vi "ConfigXMLCore.vi"(9 "ConnectionData":T1, 10 "controlsToSave":refnum<vi>[](array[refnum]), 11 "ConfigXMLControl":T2) -> ()   [LabVIEW 2016]
uses:
  ConfigXMLControl.ctl
  General/CorePluginInfo.ctl
  General/RemoteFiles/connectionData.ctl
  <vilib>/Rock Robotics/Network Tables/NT Read String.vi
panel:
  # "Core controller VI for the XML config plugin.\nhandles all saving, loading, file transfer, etc."
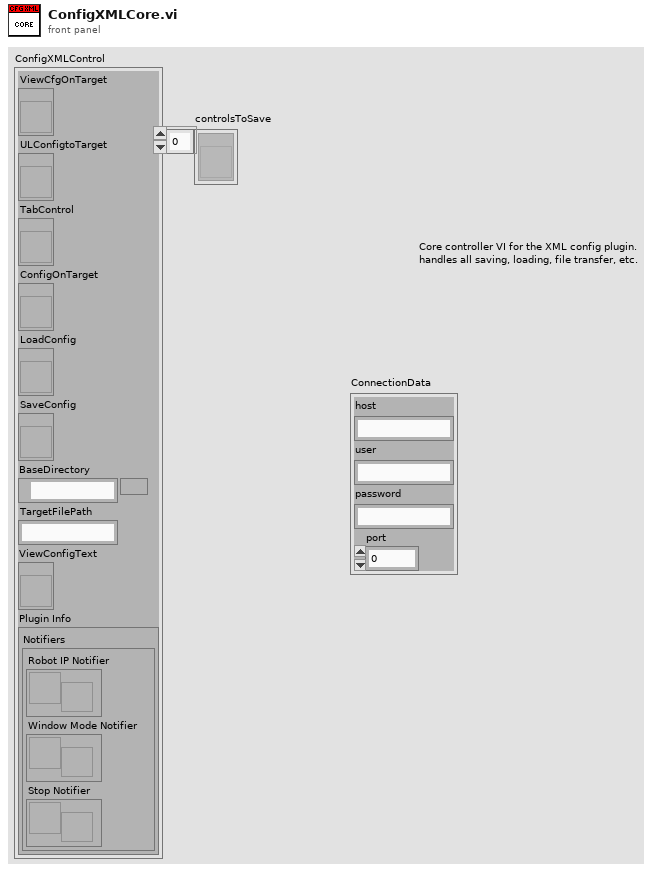
[diagram p1: front panel]
types:
  T1 = typedef "connectionData.ctl" = cluster{"host":string, "user":string, "password":string, "port":u16}
  T2 = typedef "ConfigXMLControl.ctl" = cluster{"ViewCfgOnTarget":refnum<vi>, "ULConfigtoTarget":refnum<vi>, "TabControl":refnum<vi>, "ConfigOnTarget":refnum<vi>, "LoadConfig":refnum<vi>, "SaveConfig":refnum<vi>, "BaseDirectory":path, "TargetFilePath":string, "ViewConfigText":refnum<vi>, "Plugin Info":T3}
  T3 = typedef "CorePluginInfo.ctl" = cluster{"Notifiers":cluster{"Robot IP Notifier":refnum<notifier>, "Window Mode Notifier":refnum<notifier>, "Stop Notifier":refnum<notifier>}}
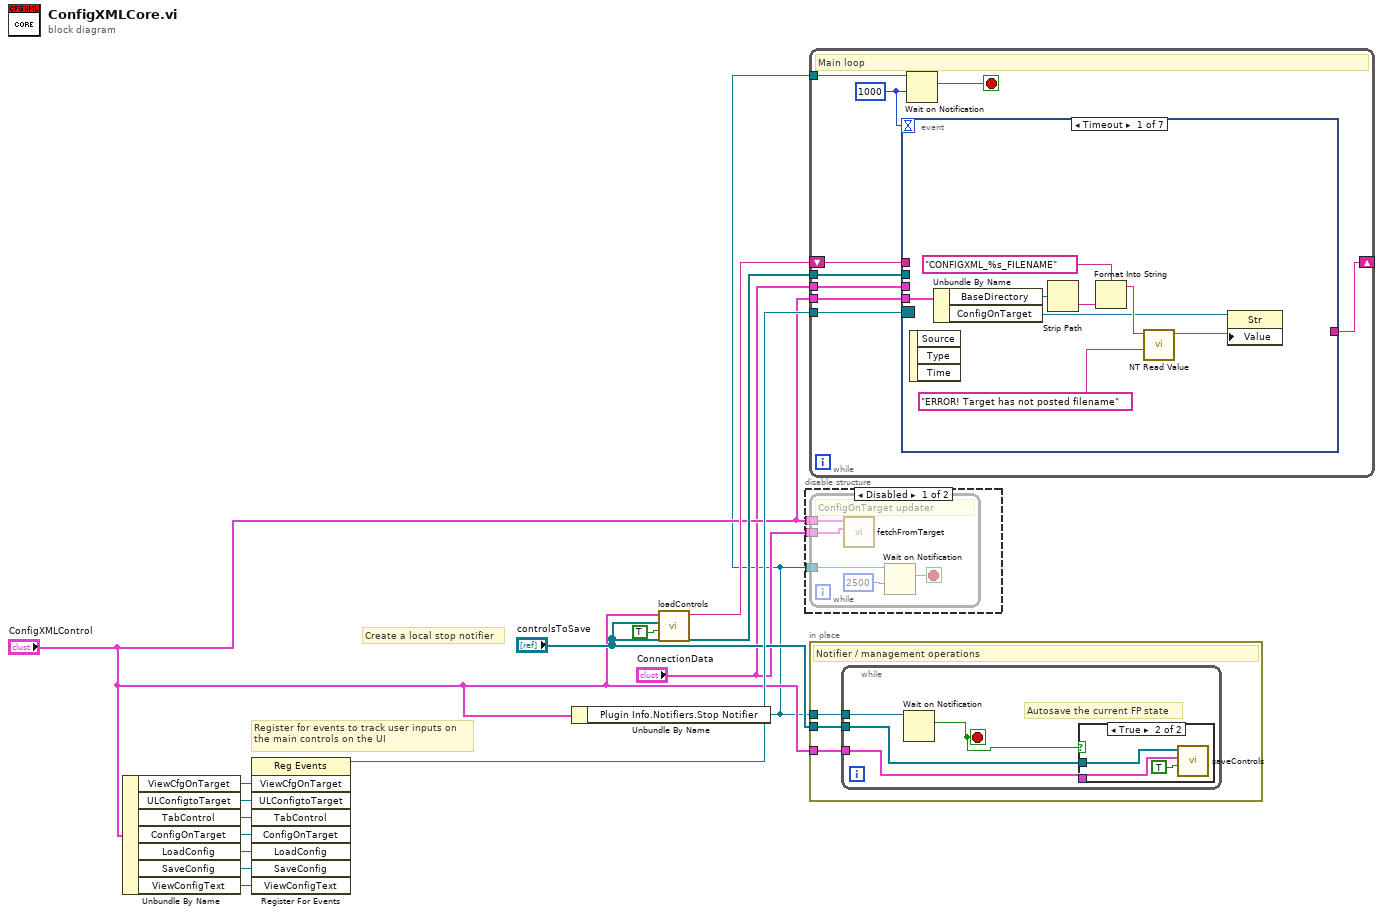
[diagram p0: block diagram]
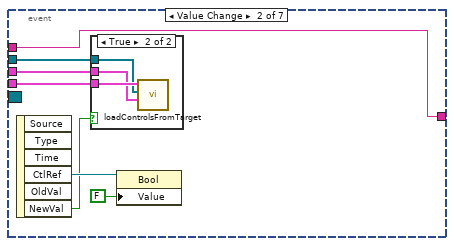
[diagram p3: hidden frame]
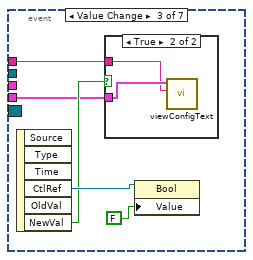
[diagram p5: hidden frame]
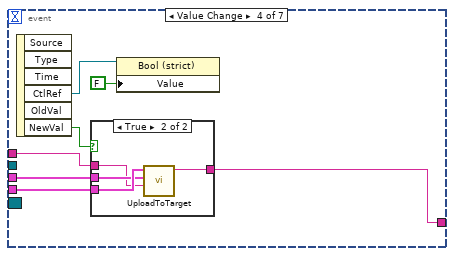
[diagram p7: hidden frame]
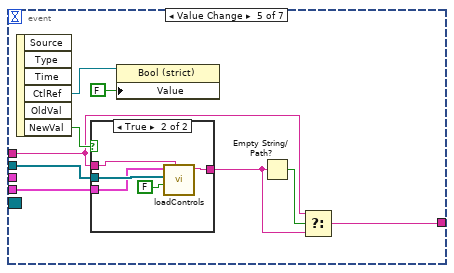
[diagram p9: hidden frame]
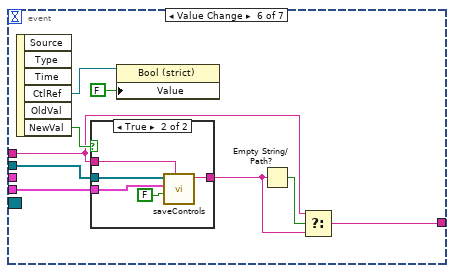
[diagram p11: hidden frame]
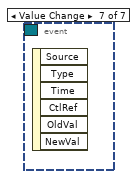
[diagram p13: hidden frame]
diagram:
  # "Create a local stop notifier"
  # "Register for events to track user inputs on\nthe main controls on the UI"
  n1 = Unbundle By Name("ConfigXMLControl") -> ("ViewCfgOnTarget"=w14:refnum<vi>, "ULConfigtoTarget"=w13:refnum<vi>, "TabControl"=w12:refnum<vi>, "ConfigOnTarget"=w11:refnum<vi>, "LoadConfig"=w10:refnum<vi>, "SaveConfig"=w9:refnum<vi>, "ViewConfigText"=w2:refnum<vi>)
  n2 = register-events(w14, w13, w12, w11, w10, w9, w2) -> (reference out=w8:refnum<event-registration>)  [unwired: 2 in, 1 out]
  n3 = Unbundle By Name("ConfigXMLControl") -> ("Plugin Info.Notifiers.Stop Notifier"=w1:refnum<notifier>)
  n4 = call "loadControls.vi"("Autoload?"=TRUE, "ControlsToLoad"="controlsToSave", "ConfigXMLControls"="ConfigXMLControl") -> ("nameUsed"=w6:string)  [unwired: 7 in, 1 out]
  n5 = disable-structure shown="Disabled" {
    disable-tunnel: "ConfigXMLControl" -> [w17 _]
    disable-tunnel: "ConnectionData" -> [w16 _]
    disable-tunnel: w1 -> [w15 _]
    frame Disabled {
      n6 = while {
        tunnel: w15 -> [w20]
        tunnel: w17 -> [w19]
        tunnel: w16 -> [w18]
        stop <- w21 stop-if-true
        # "ConfigOnTarget updater"
        n7 = call "fetchFromTarget.vi"("ConnectionData"=w18, "ConfigXMLControls"=w19) -> ()  [unwired: 5 in, 5 out]
        n8 = Wait on Notification(notifier=w20, timeout in ms (-1)=2500) -> (notification=w21:bool)  [unwired: 2 in, 3 out]
      }
    }
    frame Enabled {
    }
  }
  n9 = while {
    tunnel: w8 -> [w31]
    tunnel: "ConfigXMLControl" -> [w30]
    tunnel: "controlsToSave" -> [w29]
    tunnel: w1 -> [w27]
    shift-right: [w25] -> _
    shift-left: w6 -> [w26]
    tunnel: "ConnectionData" -> [w24]
    stop <- w28 stop-if-true
    w23 = 1000
    # "Main loop"
    n10 = event shown="[0] Timeout" {
      selector: w31 -> [_ _ _ _ _ _ _]
      dyn-events: _ -> [_ _ _ _ _ _ _]
      timeout: w23 -> [_ _ _ _ _ _ _]
      tunnel: w30 -> [w36 w43 w51 w60 w75 w88 _]
      tunnel: w29 -> [_ w41 _ _ w76 w87 _]
      tunnel: w26 -> [_ w40 w50 w58 w70 w83 _]
      tunnel: [_ w40 _ w57 w69 w84 _] -> w25
      tunnel: w24 -> [_ w42 _ w59 _ _ _]
      event Timeout {
        n11 = event-data() -> ()  [unwired: 1 in, 3 out]
        n12 = Unbundle By Name(w36) -> ("BaseDirectory"=w39:path, "ConfigOnTarget"=w33:refnum<vi>)
        n13 = Strip Path(path=w39) -> (name=w37:string)  [unwired: 1 out]
        n14 = Format Into String(format string="CONFIGXML_%s_FILENAME", w37) -> (resulting string=w35:string)  [unwired: 2 in, 1 out]
        n15 = call-poly <vilib>:"NT Read Value.vi"("Default Value"="ERROR! Target has not posted filename", "Name"=w35) -> ("String"=w32:string)  [unwired: 8 in, 1 out]
        n16 = property class="Str"(reference=w33, "Value"=w32) -> ()  [unwired: 1 in, 2 out]
      }
      event Value Change {
        n17 = event-data() -> ("CtlRef"=w45:refnum<vi>, "NewVal"=w44:bool)  [unwired: 1 in, 4 out]
        n18 = case shown="True" w44 {
          tunnel: w43 -> [_ w49]
          tunnel: w42 -> [_ w48]
          tunnel: w41 -> [_ w47]
          frame False {
          }
          frame True {
            n19 = call "loadControlsFromTarget.vi"("ConnectionData"=w48, "ControlsToLoad"=w47, "ConfigXMLControls"=w49) -> ()  [unwired: 8 in, 1 out]
          }
        }
        n20 = property class="Bool"(reference=w45, "Value"=FALSE) -> ()  [unwired: 1 in, 2 out]
      }
      event Value Change {
        n21 = event-data() -> ("CtlRef"=w54:refnum<vi>, "NewVal"=w52:bool)  [unwired: 1 in, 4 out]
        n22 = case shown="True" w52 {
          tunnel: w51 -> [_ w56]
          tunnel: w50 -> [_ w55]
          frame False {
          }
          frame True {
            n23 = call "viewConfigText.vi"("prevName"=w55, "ConfigXMLControls"=w56) -> ()  [unwired: 9 in, 1 out]
          }
        }
        n24 = property class="Bool"(reference=w54, "Value"=FALSE) -> ()  [unwired: 1 in, 2 out]
      }
      event Value Change {
        n25 = event-data() -> ("CtlRef"=w63:refnum<vi>, "NewVal"=w61:bool)  [unwired: 1 in, 4 out]
        n26 = case shown="True" w61 {
          tunnel: w60 -> [_ w68]
          tunnel: w59 -> [_ w67]
          tunnel: w58 -> [w64 w66]
          tunnel: [w64 w65] -> w57
          frame False {
          }
          frame True {
            n27 = call "UploadToTarget.vi"("previousName"=w66, "ConnectionData"=w67, "ConfigXMLControls"=w68) -> ("newName"=w65:string)  [unwired: 7 in, 1 out]
          }
        }
        n28 = property class="Bool (strict)"(reference=w63, "Value"=FALSE) -> ()  [unwired: 1 in, 2 out]
      }
      event Value Change {
        n29 = event-data() -> ("CtlRef"=w74:refnum<vi>, "NewVal"=w73:bool)  [unwired: 1 in, 4 out]
        n30 = case shown="True" w73 {
          tunnel: w75 -> [_ w80]
          tunnel: w76 -> [_ w82]
          tunnel: [_ w79] -> w71
          tunnel: w70 -> [_ w78]
          frame False {
          }
          frame True {
            n31 = call "loadControls.vi"("prevName"=w78, "Autoload?"=FALSE ("isAutoSave"), "ControlsToLoad"=w82, "ConfigXMLControls"=w80) -> ("nameUsed"=w79:string)  [unwired: 6 in, 1 out]
          }
        }
        n32 = property class="Bool (strict)"(reference=w74, "Value"=FALSE) -> ()  [unwired: 1 in, 2 out]
        n33 = Empty String/Path?(string/path=w71) -> (empty?=w72:bool)
        n34 = Select(t=w70, s=w72, f=w71) -> (s? t:f=w69:string)
      }
      event Value Change {
        n35 = event-data() -> ("CtlRef"=w91:refnum<vi>, "NewVal"=w89:bool)  [unwired: 1 in, 4 out]
        n36 = case shown="True" w89 {
          tunnel: w88 -> [_ w96]
          tunnel: w87 -> [_ w95]
          tunnel: [_ w93] -> w85
          tunnel: w83 -> [_ w92]
          frame False {
          }
          frame True {
            n37 = call "saveControls.vi"("prevName"=w92, "isAutoSave"=FALSE, "ConfigXMLControls"=w96, "ControlsToSave"=w95) -> ("nameUsed"=w93:string)  [unwired: 6 in, 1 out]
          }
        }
        n38 = property class="Bool (strict)"(reference=w91, "Value"=FALSE) -> ()  [unwired: 1 in, 2 out]
        n39 = Empty String/Path?(string/path=w85) -> (empty?=w86:bool)
        n40 = Select(t=w83, s=w86, f=w85) -> (s? t:f=w84:string)
      }
      event Value Change {
        n41 = event-data() -> ()  [unwired: 1 in, 6 out]
      }
    }
    n42 = Wait on Notification(notifier=w27, timeout in ms (-1)=w23) -> (notification=w28:bool)  [unwired: 2 in, 3 out]
  }
  n43 = in-place {
    in-place-border: w1 -> [w99]
    in-place-border: "ConfigXMLControl" -> [w98]
    in-place-border: "controlsToSave" -> [w97]
    # "Notifier / management operations"
    n44 = while {
      tunnel: w99 -> [w103]
      tunnel: w98 -> [w102]
      tunnel: w97 -> [w101]
      stop <- w100 stop-if-true
      # "Autosave the current FP state"
      n45 = Wait on Notification(notifier=w103) -> (notification=w100:bool)  [unwired: 3 in, 3 out]
      n46 = case shown="True" w100 {
        tunnel: w102 -> [_ w106]
        tunnel: w101 -> [_ w105]
        frame False {
        }
        frame True {
          n47 = call "saveControls.vi"("isAutoSave"=TRUE, "ConfigXMLControls"=w106, "ControlsToSave"=w105) -> ()  [unwired: 7 in, 2 out]
        }
      }
    }
  }
